vi "US300DepthDriver.vi"(10 "Atm Offset":dbl, 11 "Density of Water":dbl) -> (0 "error out":errorcluster, 1 "Absolute Depth (m)":dbl(slide), 2 "PSI":dbl(knob), 3 "PSI 2":dbl(graph), 4 "Actual Depth (m)":dbl(slide), 5 "Raw Voltage":dbl(graph))   [LabVIEW 2011]
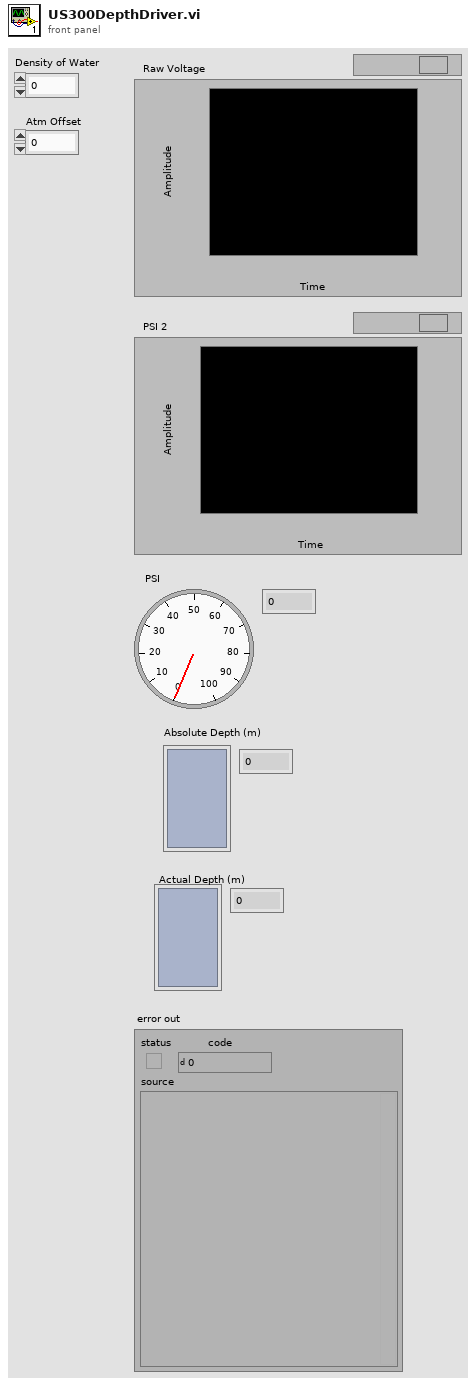
[diagram p1: front panel]
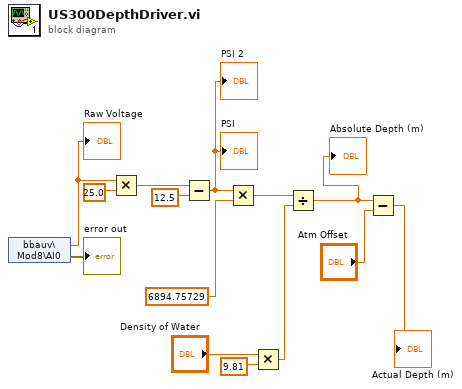
[diagram p0: block diagram]
diagram:
  n1 = shared-variable "bbauv\\Mod8\\AI0"() -> (w2:dbl, error out=→"error out":errorcluster)  [unwired: 1 in]
  "Raw Voltage" <- w2
  n2 = Multiply(x=w2, y=25.0) -> (x*y=w4:dbl)
  n3 = Subtract(x=w4, y=12.5) -> (x-y=w12:dbl)
  "PSI" <- w12
  "PSI 2" <- w12
  n4 = Multiply(x=w12, y=6894.75729) -> (x*y=w13:dbl)
  n5 = Multiply(x="Density of Water", y=9.81) -> (x*y=w8:dbl)
  n6 = Divide(x=w13, y=w8) -> (x/y=w14:dbl)
  "Absolute Depth (m)" <- w14
  n7 = Subtract(x=w14, y="Atm Offset") -> (x-y=→"Actual Depth (m)":dbl)
